vi "resample.vi"(8 "error in (no error)":errorcluster, 9 "Height":i32, 10 "Width":i32, 11 "Image in":T2) -> (0 "error out":errorcluster, 3 "Image out":T2)   [LabVIEW 2024, in "Vision.lvlib"]
uses:
  Vision.lvlib
  <vilib>/vision/Image Controls.llb/IMAQ Image.ctl
  bin/Vision.dll
panel:
  in  "Image Types Reference":T1 items=["Grayscale (U8)", "Grayscale (I16)", "Grayscale (SGL)", "Complex (CSG)", "RGB (U32)", "HSL (U32)", "RGB (U64)", "Grayscale (U16)"]
  out "return type":i32
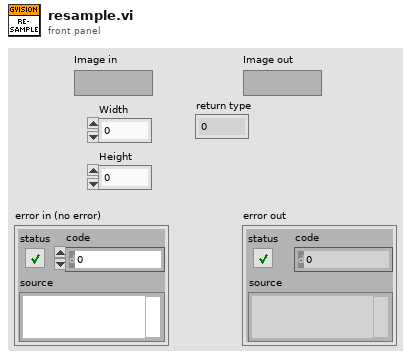
[diagram p1: front panel]
types:
  T1 = typedef "Image Type" = u32
  T2 = typedef "IMAQ Image.ctl" = refnum<image>
  T3 = enum32{"Map Pixel Pointer", "Unmap Pixel Pointer", "Get Pixels Infos"}
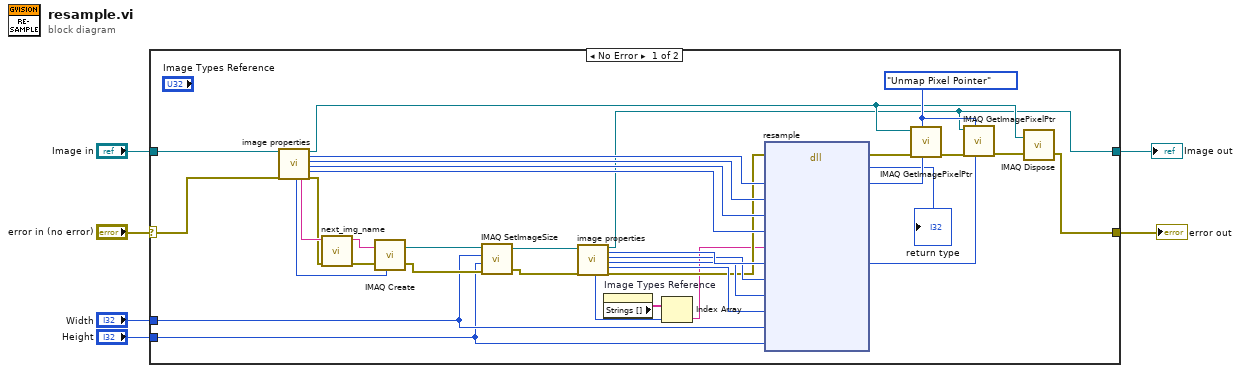
[diagram p0: block diagram]
diagram:
  n1 = case shown="No Error" "error in (no error)" {
    selector: "error in (no error)" -> [w12 w43]
    tunnel: "Image in" -> [w13 w42]
    tunnel: [w41 w43] -> w4
    tunnel: [w18 w42] -> w3
    tunnel: "Width" -> [w26 _]
    tunnel: "Height" -> [w25 _]
    frame No Error {
      w37 = T3."Unmap Pixel Pointer" ("Function")
      n2 = call "image properties.vi"("Image in"=w13, "error in (no error)"=w12) -> ("Image Type"=w11:T1, "Image Name"=w17:string, "Image out"=w21:T2, "Pixel Pointer out"=w36:u64, "Line Width"=w35:i32, "X Resolution"=w34:i32, "Y Resolution"=w33:i32, "error out"=w16:errorcluster)  [unwired: 10 in]
      n3 = call "next_img_name.vi"("error in (no error)"=w16, "name in"=w17) -> ("error out"=w15:errorcluster, "name out"=w14:string)  [unwired: 8 in]
      n4 = call "IMAQ Create"("Image Name"=w14, "Image Type"=w11, "error in (no error)"=w15) -> ("New Image"=w28:T2, "error out"=w27:errorcluster)  [unwired: 2 in]
      n5 = call "IMAQ SetImageSize"("error in (no error)"=w27, "Y Resolution"=w25, "X Resolution"=w26, "Image"=w28) -> ("error out"=w23:errorcluster, "Image Out"=w24:T2)  [unwired: 1 in]
      n6 = call "image properties.vi"("Image in"=w24, "error in (no error)"=w23) -> ("Image Type"=w8:T1, "Image out"=w18:T2, "Pixel Pointer out"=w32:u64, "Line Width"=w31:i32, "X Resolution"=w30:i32, "Y Resolution"=w29:i32, "error out"=w22:errorcluster)  [unwired: 10 in, 1 out]
      n7 = property on="Image Types Reference" class="Ring (strict)"() -> ("Strings []"=w9:string[])  [unwired: 2 in, 2 out]
      n8 = Index Array(array=w9, index=w8) -> (element=w7:string)
      n9 = dll-call lib="C:/Users/cfang/Desktop/nebraska-silicon-lab/pixel-gantry-control/Gantry/Shared Components/bin/Vision.dll" fn="resample"(error in=w22, "src_imgPtr"=w36, "src_imgLineWidth"=w35, "src_imgWidth"=w34, "src_imgHeight"=w33, "src_type"=w7, "dst_imgPtr"=w32, "dst_imgLineWidth"=w31, "dst_imgWidth"=w30, "dst_imgHeight"=w29, "new_width"=w26, "new_height"=w25) -> (error out=w39:errorcluster, "return type"=→"return type":i32, "src_imgPtr"=w20:u64, "dst_imgPtr"=w19:u64)  [unwired: 11 in, 1 out]
      n10 = call "IMAQ GetImagePixelPtr"("Pixel Pointer in"=w20, "Function"=w37, "error in (no error)"=w39, "Image"=w21) -> ("error out"=w40:errorcluster)  [unwired: 2 in, 5 out]
      n11 = call "IMAQ GetImagePixelPtr"("Pixel Pointer in"=w19, "Function"=w37, "error in (no error)"=w40, "Image"=w18) -> ("error out"=w38:errorcluster)  [unwired: 2 in, 5 out]
      n12 = call "IMAQ Dispose"("Image"=w21, "error in (no error)"=w38) -> ("error out"=w41:errorcluster)  [unwired: 4 in]
    }
    frame Error {
    }
  }
  "Image out" <- w3
  "error out" <- w4
